vi "Write error.vi"(8 "error in (no error)":errorcluster, 10 "error":errorcluster, 11 "Error Report in":refnum<class "Error Report.lvclass">) -> (0 "error out":errorcluster, 3 "Error Report out":refnum<class "Error Report.lvclass">)   [LabVIEW 2016, in "Controller API.lvlib" / "Error Result.lvlib" / "Error Report.lvclass"]
uses:
  Error Report.lvclass
  Error Report.lvclass/Error Report.ctl
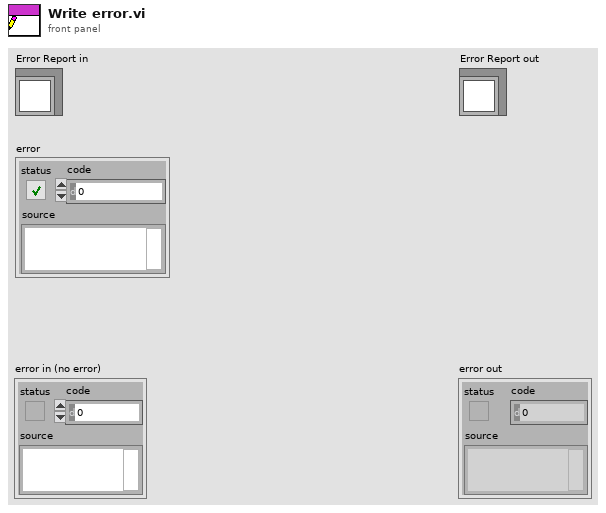
[diagram p1: front panel]
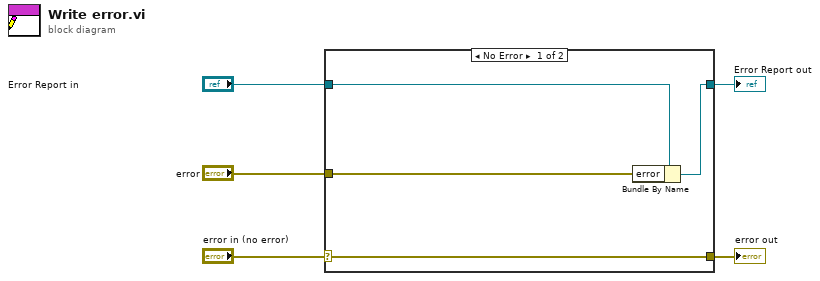
[diagram p0: block diagram]
diagram:
  n1 = case shown="No Error" "error in (no error)" {
    selector: "error in (no error)" -> [w9 w10]
    tunnel: [w9 w10] -> w4
    tunnel: [w7 w11] -> w2
    tunnel: "Error Report in" -> [w8 w11]
    tunnel: "error" -> [w6 _]
    frame No Error {
      n2 = Bundle By Name(cluster=w8, "error"=w6) -> (w7:refnum<class "Error Report.lvclass">)
    }
    frame Error {
    }
  }
  "error out" <- w4
  "Error Report out" <- w2
